vi "MH_T2HeaderInfo.vi"(8 "entrée d'erreur":errorcluster, 10 "CountRates":i32[](array[numeric]), 11 "InstrClass":refnum<class "MultiHarp150.lvclass"> caption="DNL_LabVIEW Object in") -> (0 "sortie d'erreur":errorcluster, 2 "HeaderTags":T1(array[cluster]))   [LabVIEW 2019, in "MultiHarp150.lvclass"]
uses:
  MultiHarp150.lvclass
  MultiHarp150.lvclass/MultiHarp150.ctl
panel:
  in  "BaseTagArray":T1(array[cluster])=[{"TagIdent"="File_GUID", "TagIndex"=-1, "TagType"=1073872895, "TagValue"=40, "TagAuxData"="{197B8EE0-02FE-45EA-A6B5-3F8BBDE2D882}\u0000\u0000"}, {"TagIdent"="File_AssuredContent", "TagIndex"=-1, "TagType"=1073872895, "TagValue"=32, "TagAuxData"="MultiHarp: HWSETG SWSETG\u0000\u0000\u0000\u0000\u0000\u0000\u0000\u0000"}, {"TagIdent"="CreatorSW_ContentVersion", "TagIndex"=-1, "TagType"=1073872895, "TagValue"=8, "TagAuxData"="1.0\u0000\u0000\u0000\u0000\u0000"}, {"TagIdent"="CreatorSW_Name", "TagIndex"=-1, "TagType"=1073872895, "TagValue"=16, "TagAuxData"="MultiHarp AcqUI\u0000"}, {"TagIdent"="CreatorSW_Version", "TagIndex"=-1, "TagType"=1073872895, "TagValue"=8, "TagAuxData"="3.0.0.0\u0000"}, {"TagIdent"="File_CreatingTime", "TagIndex"=-1, "TagType"=553648136, "TagValue"=4676398420989345414, "TagAuxData"=""}, {"TagIdent"="File_Comment", "TagIndex"=-1, "TagType"=1073872895, "TagValue"=8, "TagAuxData"="T2 Mode\u0000"}, {"TagIdent"="Measurement_Mode", "TagIndex"=-1, "TagType"=268435464, "TagValue"=2, "TagAuxData"=""}, {"TagIdent"="Measurement_SubMode", "TagIndex"=-1, "TagType"=268435464, "TagValue"=0, "TagAuxData"=""}, {"TagIdent"="TTResult_StopReason", "TagIndex"=-1, "TagType"=268435464, "TagValue"=0, "TagAuxData"=""}, {"TagIdent"="Fast_Load_End", "TagIndex"=-1, "TagType"=-65528, "TagValue"=0, "TagAuxData"=""}, {"TagIdent"="TTResultFormat_TTTRRecType", "TagIndex"=-1, "TagType"=268435464, "TagValue"=66055, "TagAuxData"=""}, {"TagIdent"="TTResultFormat_BitsPerRecord", "TagIndex"=-1, "TagType"=268435464, "TagValue"=32, "TagAuxData"=""}, {"TagIdent"="MeasDesc_BinningFactor", "TagIndex"=-1, "TagType"=268435464, "TagValue"=32, "TagAuxData"=""}, {"TagIdent"="MeasDesc_Offset", "TagIndex"=-1, "TagType"=268435464, "TagValue"=0, "TagAuxData"=""}, {"TagIdent"="MeasDesc_AcquisitionTime", "TagIndex"=-1, "TagType"=268435464, "TagValue"=900000, "TagAuxData"=""}, {"TagIdent"="MeasDesc_StopAt", "TagIndex"=-1, "TagType"=268435464, "TagValue"=4294967295, "TagAuxData"=""}, {"TagIdent"="MeasDesc_StopOnOvfl", "TagIndex"=-1, "TagType"=8, "TagValue"=0, "TagAuxData"=""}, {"TagIdent"="MeasDesc_Restart", "TagIndex"=-1, "TagType"=8, "TagValue"=0, "TagAuxData"=""}, {"TagIdent"="CurSWSetting_DispLog", "TagIndex"=-1, "TagType"=8, "TagValue"=-1, "TagAuxData"=""}, {"TagIdent"="CurSWSetting_DispAxisTimeFrom", "TagIndex"=-1, "TagType"=268435464, "TagValue"=1, "TagAuxData"=""}, {"TagIdent"="CurSWSetting_DispAxisTimeTo", "TagIndex"=-1, "TagType"=268435464, "TagValue"=120, "TagAuxData"=""}, {"TagIdent"="CurSWSetting_DispAxisCountFrom", "TagIndex"=-1, "TagType"=268435464, "TagValue"=1, "TagAuxData"=""}, {"TagIdent"="CurSWSetting_DispAxisCountTo", "TagIndex"=-1, "TagType"=268435464, "TagValue"=10000, "TagAuxData"=""}, {"TagIdent"="CurSWSetting_DispCurves", "TagIndex"=-1, "TagType"=268435464, "TagValue"=16, "TagAuxData"=""}, {"TagIdent"="CurSWSetting_DispCurve_MapTo", "TagIndex"=0, "TagType"=268435464, "TagValue"=0, "TagAuxData"=""}, {"TagIdent"="CurSWSetting_DispCurve_Show", "TagIndex"=0, "TagType"=8, "TagValue"=-1, "TagAuxData"=""}, {"TagIdent"="CurSWSetting_DispCurve_MapTo", "TagIndex"=1, "TagType"=268435464, "TagValue"=1, "TagAuxData"=""}, {"TagIdent"="CurSWSetting_DispCurve_Show", "TagIndex"=1, "TagType"=8, "TagValue"=-1, "TagAuxData"=""}, {"TagIdent"="CurSWSetting_DispCurve_MapTo", "TagIndex"=2, "TagType"=268435464, "TagValue"=2, "TagAuxData"=""}, {"TagIdent"="CurSWSetting_DispCurve_Show", "TagIndex"=2, "TagType"=8, "TagValue"=-1, "TagAuxData"=""}, {"TagIdent"="CurSWSetting_DispCurve_MapTo", "TagIndex"=3, "TagType"=268435464, "TagValue"=3, "TagAuxData"=""}, {"TagIdent"="CurSWSetting_DispCurve_Show", "TagIndex"=3, "TagType"=8, "TagValue"=-1, "TagAuxData"=""}, {"TagIdent"="CurSWSetting_DispCurve_MapTo", "TagIndex"=4, "TagType"=268435464, "TagValue"=4, "TagAuxData"=""}, {"TagIdent"="CurSWSetting_DispCurve_Show", "TagIndex"=4, "TagType"=8, "TagValue"=-1, "TagAuxData"=""}, {"TagIdent"="CurSWSetting_DispCurve_MapTo", "TagIndex"=5, "TagType"=268435464, "TagValue"=5, "TagAuxData"=""}, {"TagIdent"="CurSWSetting_DispCurve_Show", "TagIndex"=5, "TagType"=8, "TagValue"=-1, "TagAuxData"=""}, {"TagIdent"="CurSWSetting_DispCurve_MapTo", "TagIndex"=6, "TagType"=268435464, "TagValue"=6, "TagAuxData"=""}, {"TagIdent"="CurSWSetting_DispCurve_Show", "TagIndex"=6, "TagType"=8, "TagValue"=-1, "TagAuxData"=""}, {"TagIdent"="CurSWSetting_DispCurve_MapTo", "TagIndex"=7, "TagType"=268435464, "TagValue"=7, "TagAuxData"=""}, {"TagIdent"="CurSWSetting_DispCurve_Show", "TagIndex"=7, "TagType"=8, "TagValue"=-1, "TagAuxData"=""}, {"TagIdent"="CurSWSetting_DispCurve_MapTo", "TagIndex"=8, "TagType"=268435464, "TagValue"=8, "TagAuxData"=""}, {"TagIdent"="CurSWSetting_DispCurve_Show", "TagIndex"=8, "TagType"=8, "TagValue"=-1, "TagAuxData"=""}, {"TagIdent"="CurSWSetting_DispCurve_MapTo", "TagIndex"=9, "TagType"=268435464, "TagValue"=9, "TagAuxData"=""}, {"TagIdent"="CurSWSetting_DispCurve_Show", "TagIndex"=9, "TagType"=8, "TagValue"=-1, "TagAuxData"=""}, {"TagIdent"="CurSWSetting_DispCurve_MapTo", "TagIndex"=10, "TagType"=268435464, "TagValue"=10, "TagAuxData"=""}, {"TagIdent"="CurSWSetting_DispCurve_Show", "TagIndex"=10, "TagType"=8, "TagValue"=-1, "TagAuxData"=""}, {"TagIdent"="CurSWSetting_DispCurve_MapTo", "TagIndex"=11, "TagType"=268435464, "TagValue"=11, "TagAuxData"=""}, {"TagIdent"="CurSWSetting_DispCurve_Show", "TagIndex"=11, "TagType"=8, "TagValue"=-1, "TagAuxData"=""}, {"TagIdent"="CurSWSetting_DispCurve_MapTo", "TagIndex"=12, "TagType"=268435464, "TagValue"=12, "TagAuxData"=""}, {"TagIdent"="CurSWSetting_DispCurve_Show", "TagIndex"=12, "TagType"=8, "TagValue"=-1, "TagAuxData"=""}, {"TagIdent"="CurSWSetting_DispCurve_MapTo", "TagIndex"=13, "TagType"=268435464, "TagValue"=13, "TagAuxData"=""}, {"TagIdent"="CurSWSetting_DispCurve_Show", "TagIndex"=13, "TagType"=8, "TagValue"=-1, "TagAuxData"=""}, {"TagIdent"="CurSWSetting_DispCurve_MapTo", "TagIndex"=14, "TagType"=268435464, "TagValue"=14, "TagAuxData"=""}, {"TagIdent"="CurSWSetting_DispCurve_Show", "TagIndex"=14, "TagType"=8, "TagValue"=-1, "TagAuxData"=""}, {"TagIdent"="CurSWSetting_DispCurve_MapTo", "TagIndex"=15, "TagType"=268435464, "TagValue"=15, "TagAuxData"=""}, {"TagIdent"="CurSWSetting_DispCurve_Show", "TagIndex"=15, "TagType"=8, "TagValue"=-1, "TagAuxData"=""}, {"TagIdent"="HW_Type", "TagIndex"=-1, "TagType"=1073872895, "TagValue"=24, "TagAuxData"="MultiHarp 150 4P\u0000\u0000\u0000\u0000\u0000\u0000\u0000\u0000"}, {"TagIdent"="HW_PartNo", "TagIndex"=-1, "TagType"=1073872895, "TagValue"=8, "TagAuxData"="930043\u0000\u0000"}, {"TagIdent"="HW_Version", "TagIndex"=-1, "TagType"=1073872895, "TagValue"=8, "TagAuxData"="1.0\u0000\u0000\u0000\u0000\u0000"}, {"TagIdent"="HW_SerialNo", "TagIndex"=-1, "TagType"=1073872895, "TagValue"=8, "TagAuxData"="1043897\u0000"}, {"TagIdent"="HW_Features", "TagIndex"=-1, "TagType"=285212680, "TagValue"=183, "TagAuxData"=""}, {"TagIdent"="HW_BaseResolution", "TagIndex"=-1, "TagType"=536870920, "TagValue"=4437731733528994965, "TagAuxData"=""}, {"TagIdent"="HW_InpChannels", "TagIndex"=-1, "TagType"=268435464, "TagValue"=4, "TagAuxData"=""}, {"TagIdent"="HW_ExternalRefClock", "TagIndex"=-1, "TagType"=8, "TagValue"=0, "TagAuxData"=""}, {"TagIdent"="HW_ExternalDevices", "TagIndex"=-1, "TagType"=268435464, "TagValue"=0, "TagAuxData"=""}, {"TagIdent"="HWTriggerOut_Period", "TagIndex"=-1, "TagType"=536870920, "TagValue"=4502148214488346441, "TagAuxData"=""}, {"TagIdent"="HWTriggerOut_On", "TagIndex"=-1, "TagType"=8, "TagValue"=0, "TagAuxData"=""}, {"TagIdent"="HW_InputHysteresis", "TagIndex"=-1, "TagType"=8, "TagValue"=0, "TagAuxData"=""}, {"TagIdent"="HWSync_Divider", "TagIndex"=-1, "TagType"=268435464, "TagValue"=1, "TagAuxData"=""}, {"TagIdent"="HWSync_TrgLevel", "TagIndex"=-1, "TagType"=268435464, "TagValue"=-10, "TagAuxData"=""}, {"TagIdent"="HWSync_TrgEdge", "TagIndex"=-1, "TagType"=268435464, "TagValue"=0, "TagAuxData"=""}, {"TagIdent"="HWSync_Offset", "TagIndex"=-1, "TagType"=268435464, "TagValue"=27000, "TagAuxData"=""}, {"TagIdent"="HWSync_TdCode", "TagIndex"=-1, "TagType"=268435464, "TagValue"=0, "TagAuxData"=""}, {"TagIdent"="HWInpChan_TrgLevel", "TagIndex"=0, "TagType"=268435464, "TagValue"=-150, "TagAuxData"=""}, {"TagIdent"="HWInpChan_TrgEdge", "TagIndex"=0, "TagType"=268435464, "TagValue"=0, "TagAuxData"=""}, {"TagIdent"="HWInpChan_Offset", "TagIndex"=0, "TagType"=268435464, "TagValue"=0, "TagAuxData"=""}, {"TagIdent"="HWInpChan_Enabled", "TagIndex"=0, "TagType"=8, "TagValue"=-1, "TagAuxData"=""}, {"TagIdent"="HWInpChan_TdCode", "TagIndex"=0, "TagType"=268435464, "TagValue"=0, "TagAuxData"=""}, {"TagIdent"="HWInpChan_TrgLevel", "TagIndex"=1, "TagType"=268435464, "TagValue"=-150, "TagAuxData"=""}, {"TagIdent"="HWInpChan_TrgEdge", "TagIndex"=1, "TagType"=268435464, "TagValue"=0, "TagAuxData"=""}, {"TagIdent"="HWInpChan_Offset", "TagIndex"=1, "TagType"=268435464, "TagValue"=0, "TagAuxData"=""}, {"TagIdent"="HWInpChan_Enabled", "TagIndex"=1, "TagType"=8, "TagValue"=-1, "TagAuxData"=""}, {"TagIdent"="HWInpChan_TdCode", "TagIndex"=1, "TagType"=268435464, "TagValue"=0, "TagAuxData"=""}, {"TagIdent"="HWInpChan_TrgLevel", "TagIndex"=2, "TagType"=268435464, "TagValue"=-50, "TagAuxData"=""}, {"TagIdent"="HWInpChan_TrgEdge", "TagIndex"=2, "TagType"=268435464, "TagValue"=0, "TagAuxData"=""}, {"TagIdent"="HWInpChan_Offset", "TagIndex"=2, "TagType"=268435464, "TagValue"=0, "TagAuxData"=""}, {"TagIdent"="HWInpChan_Enabled", "TagIndex"=2, "TagType"=8, "TagValue"=-1, "TagAuxData"=""}, {"TagIdent"="HWInpChan_TdCode", "TagIndex"=2, "TagType"=268435464, "TagValue"=0, "TagAuxData"=""}, {"TagIdent"="HWInpChan_TrgLevel", "TagIndex"=3, "TagType"=268435464, "TagValue"=-50, "TagAuxData"=""}, {"TagIdent"="HWInpChan_TrgEdge", "TagIndex"=3, "TagType"=268435464, "TagValue"=0, "TagAuxData"=""}, {"TagIdent"="HWInpChan_Offset", "TagIndex"=3, "TagType"=268435464, "TagValue"=0, "TagAuxData"=""}, {"TagIdent"="HWInpChan_Enabled", "TagIndex"=3, "TagType"=8, "TagValue"=-1, "TagAuxData"=""}, {"TagIdent"="HWInpChan_TdCode", "TagIndex"=3, "TagType"=268435464, "TagValue"=0, "TagAuxData"=""}, {"TagIdent"="MeasDesc_Resolution", "TagIndex"=-1, "TagType"=536870920, "TagValue"=4437731733528994965, "TagAuxData"=""}, {"TagIdent"="HW_Markers", "TagIndex"=-1, "TagType"=268435464, "TagValue"=4, "TagAuxData"=""}, {"TagIdent"="HWMarkers_RisingEdge", "TagIndex"=0, "TagType"=8, "TagValue"=0, "TagAuxData"=""}, {"TagIdent"="HWMarkers_RisingEdge", "TagIndex"=1, "TagType"=8, "TagValue"=0, "TagAuxData"=""}, {"TagIdent"="HWMarkers_RisingEdge", "TagIndex"=2, "TagType"=8, "TagValue"=0, "TagAuxData"=""}, {"TagIdent"="HWMarkers_RisingEdge", "TagIndex"=3, "TagType"=8, "TagValue"=0, "TagAuxData"=""}, {"TagIdent"="HWMarkers_Enabled", "TagIndex"=0, "TagType"=8, "TagValue"=-1, "TagAuxData"=""}, {"TagIdent"="HWMarkers_Enabled", "TagIndex"=1, "TagType"=8, "TagValue"=-1, "TagAuxData"=""}, {"TagIdent"="HWMarkers_Enabled", "TagIndex"=2, "TagType"=8, "TagValue"=-1, "TagAuxData"=""}, {"TagIdent"="HWMarkers_Enabled", "TagIndex"=3, "TagType"=8, "TagValue"=-1, "TagAuxData"=""}, {"TagIdent"="HWMarkers_HoldOff", "TagIndex"=-1, "TagType"=268435464, "TagValue"=0, "TagAuxData"=""}, {"TagIdent"="MeasDesc_GlobalResolution", "TagIndex"=-1, "TagType"=536870920, "TagValue"=4437731733528994965, "TagAuxData"=""}, {"TagIdent"="TTResult_SyncRate", "TagIndex"=-1, "TagType"=268435464, "TagValue"=0, "TagAuxData"=""}, {"TagIdent"="TTResult_InputRate", "TagIndex"=0, "TagType"=268435464, "TagValue"=9126, "TagAuxData"=""}, {"TagIdent"="TTResult_InputRate", "TagIndex"=1, "TagType"=268435464, "TagValue"=8247, "TagAuxData"=""}, {"TagIdent"="TTResult_InputRate", "TagIndex"=2, "TagType"=268435464, "TagValue"=0, "TagAuxData"=""}, {"TagIdent"="TTResult_InputRate", "TagIndex"=3, "TagType"=268435464, "TagValue"=0, "TagAuxData"=""}, {"TagIdent"="TTResult_StopAfter", "TagIndex"=-1, "TagType"=268435464, "TagValue"=900000, "TagAuxData"=""}, {"TagIdent"="TTResult_NumberOfRecords", "TagIndex"=-1, "TagType"=268435464, "TagValue"=10000, "TagAuxData"=""}, {"TagIdent"="TTResult_MDescWarningFlags", "TagIndex"=-1, "TagType"=285212680, "TagValue"=0, "TagAuxData"=""}, {"TagIdent"="Header_End", "TagIndex"=-1, "TagType"=-65528, "TagValue"=0, "TagAuxData"=""}] {"TagType" format="%x"}
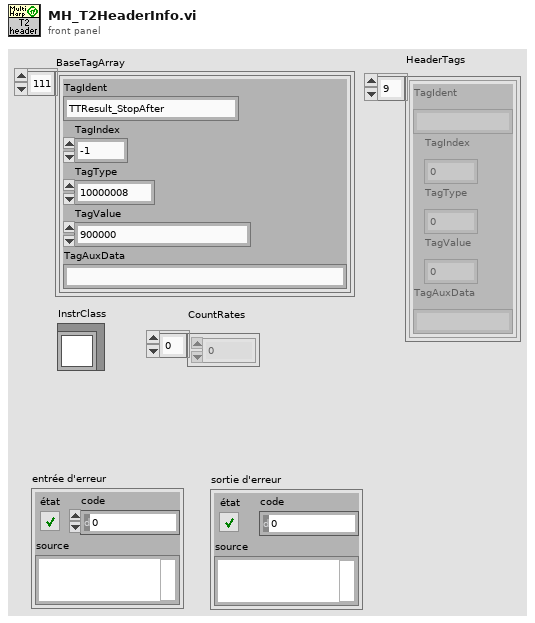
[diagram p1: front panel]
types:
  T1 = cluster{"TagIdent":string, "TagIndex":i32, "TagType":i32, "TagValue":i64, "TagAuxData":string}[]
  T2 = cluster{"TagIdent":string, "TagIndex":i32, "TagType":i32, "TagValue":i64, "TagAuxData":string}
  T3 = enum16{"5", "10", "20", "40", "80", "160", "320", "640", "1280", "2560", "5120", "10240", "20480", "40960", "81920", "163840", "327680", "655360", "1310720", "2621440", "5242880", "10485760", "20971520", "41943040"}
  T4 = typedef "MH_InputChannel_LS.ctl" = cluster{"Name":string, "Enable":bool, "Edge":i32, "Level":i32, "Offset":i32, "UseDeadTime":bool, "DeadTime":i32}
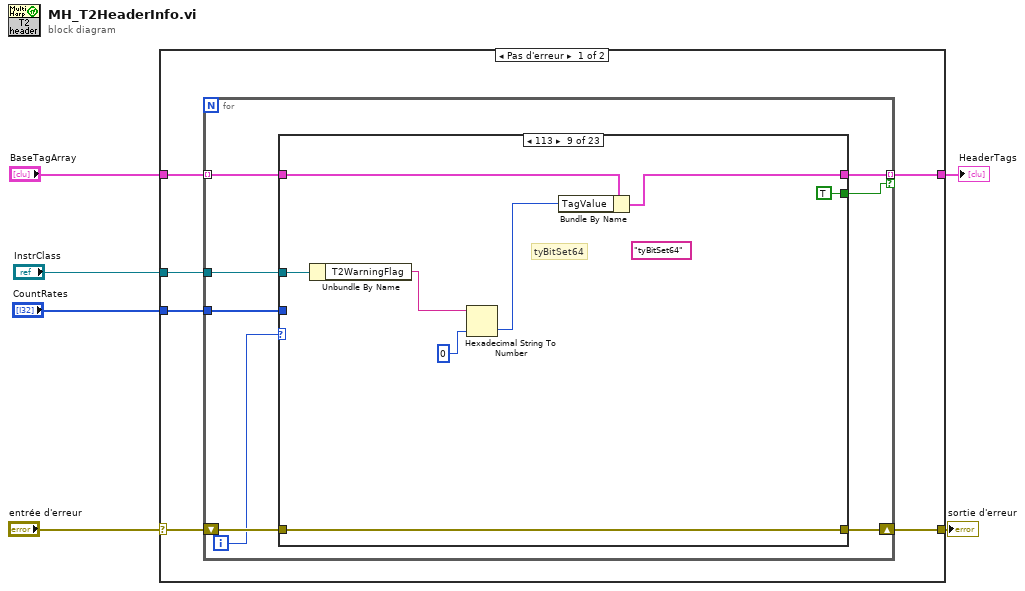
[diagram p0: block diagram]
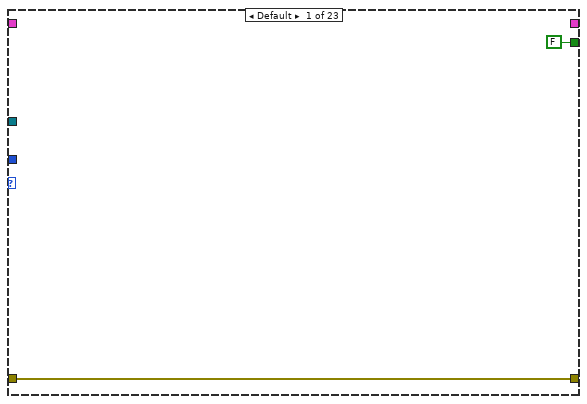
[diagram p2: hidden frame]
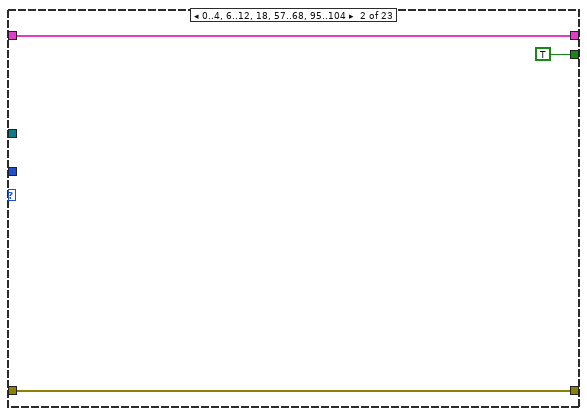
[diagram p3: hidden frame]
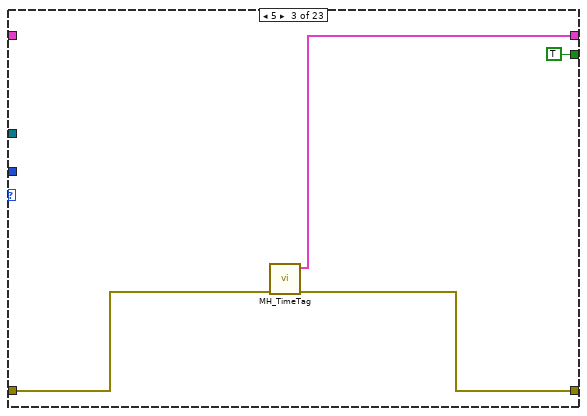
[diagram p4: hidden frame]
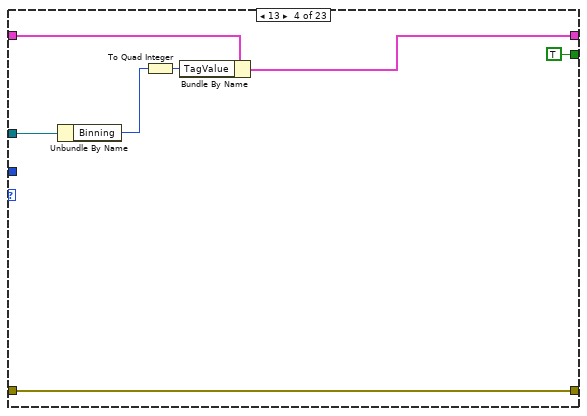
[diagram p5: hidden frame]
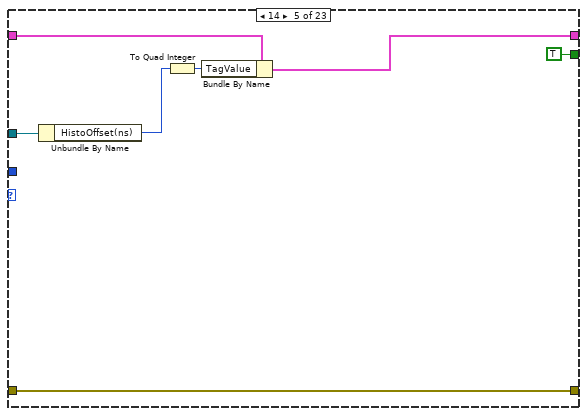
[diagram p6: hidden frame]
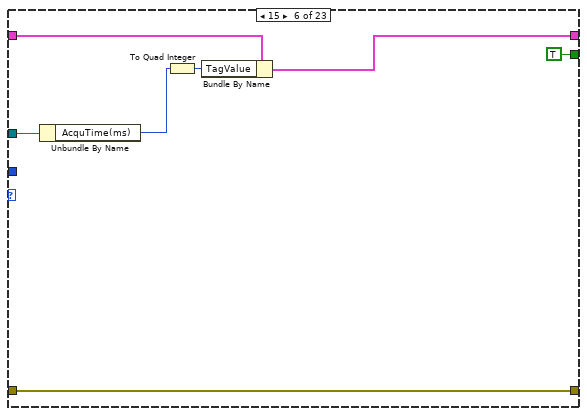
[diagram p7: hidden frame]
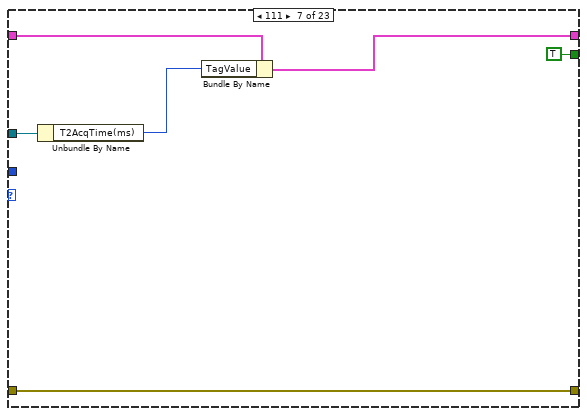
[diagram p8: hidden frame]
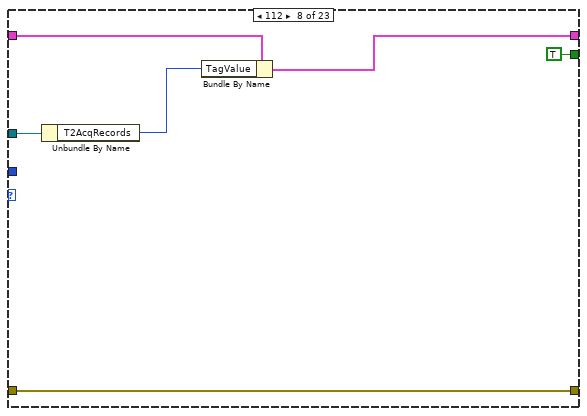
[diagram p9: hidden frame]
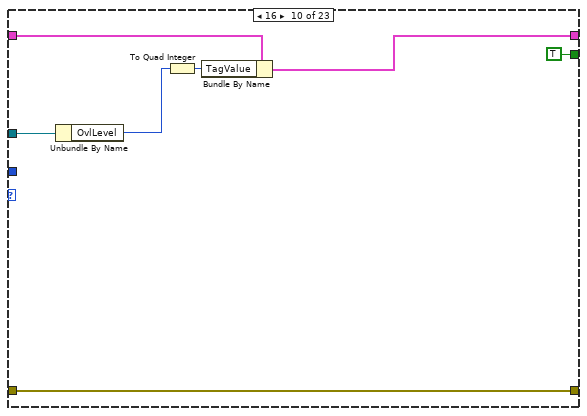
[diagram p10: hidden frame]
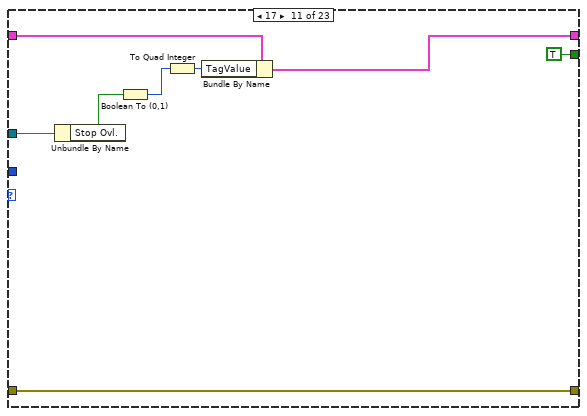
[diagram p11: hidden frame]
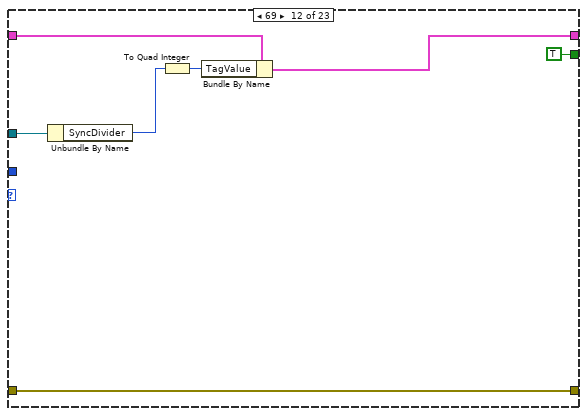
[diagram p12: hidden frame]
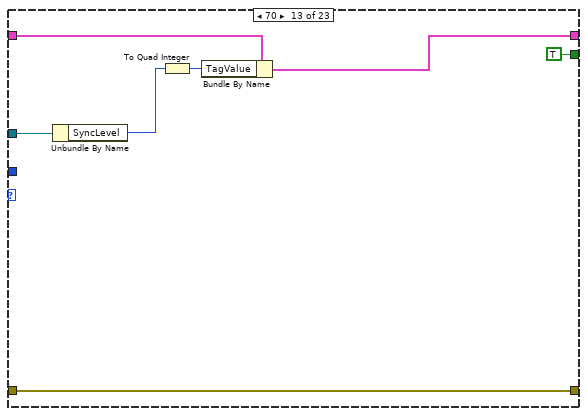
[diagram p13: hidden frame]
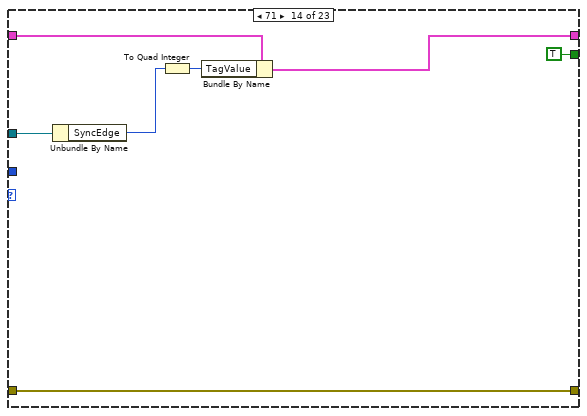
[diagram p14: hidden frame]
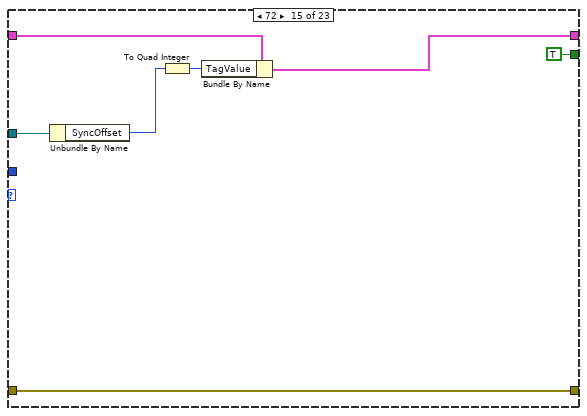
[diagram p15: hidden frame]
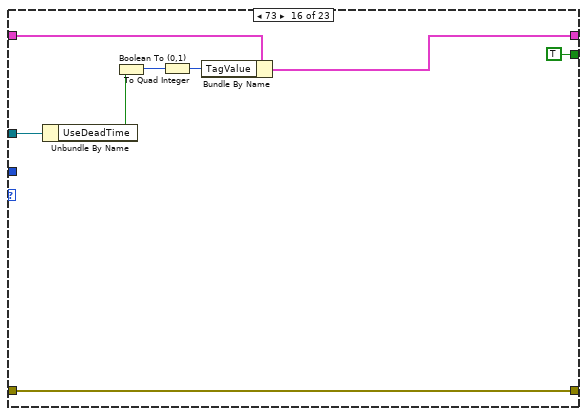
[diagram p16: hidden frame]
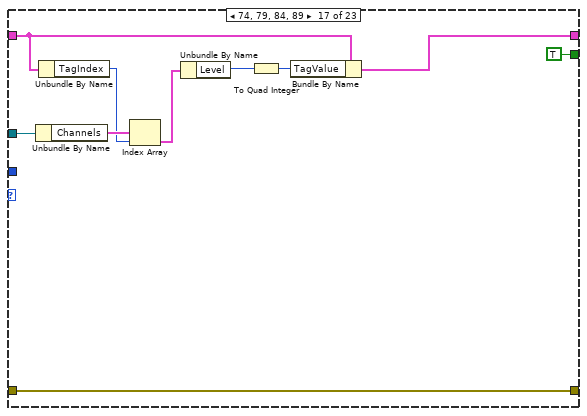
[diagram p17: hidden frame]
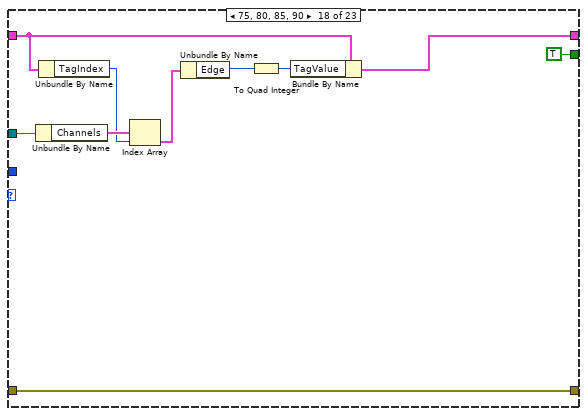
[diagram p18: hidden frame]
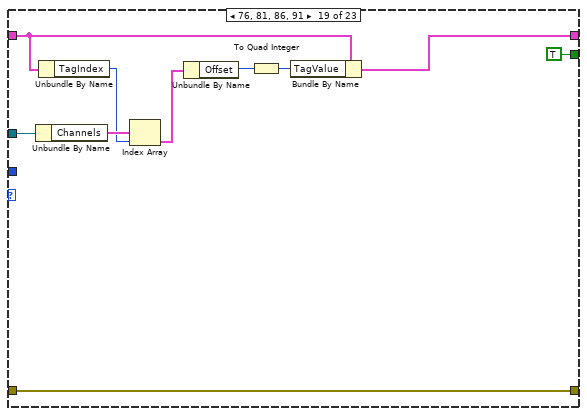
[diagram p19: hidden frame]
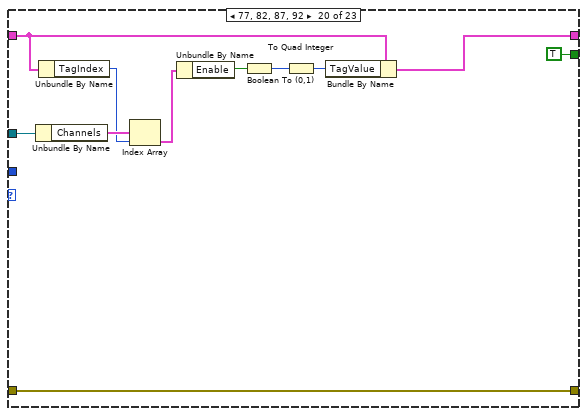
[diagram p20: hidden frame]
diagram:
  n1 = case shown="Pas d'erreur" "entrée d'erreur" {
    selector: "entrée d'erreur" -> [w11 w198]
    tunnel: [w12 w198] -> w6
    tunnel: "BaseTagArray" -> [w10 _]
    tunnel: "InstrClass" -> [w9 _]
    tunnel: [w8 _] -> w2
    tunnel: "CountRates" -> [w7 _]
    frame No Error {
      n2 = for {
        shift-right: [w20] -> w12
        shift-left: w11 -> [w19]
        tunnel: w10 -> [w14] mode=indexing
        tunnel: [w17] -> w8 mode=indexing if=w15
        tunnel: w9 -> [w16]
        tunnel: w7 -> [w13]
        i -> [w18]
        n3 = case shown="113" w18 {
          selector: w18 -> [_ _ _ _ _ _ _ _ _ _ _ _ _ _ _ _ _ _ _ _ _ _ w190]
          tunnel: [w22 w24 w29 w31 w38 w46 w53 w59 w67 w72 w81 w88 w95 w102 w109 w117 w128 w138 w148 w159 w170 w185 w196] -> w20
          tunnel: w19 -> [w22 w24 w28 w31 w38 w46 w53 w59 w67 w72 w81 w88 w95 w102 w109 w117 w128 w138 w148 w159 w170 w185 w196]
          tunnel: w14 -> [_ w25 _ w35 w42 w49 w55 w61 w69 w76 w84 w91 w98 w105 w112 w120 w123 w133 w143 w154 w165 w183 w194]
          tunnel: [_ w25 w27 w33 w40 w48 w54 w60 w68 w74 w83 w90 w97 w104 w111 w119 w130 w140 w150 w161 w172 w186 w197] -> w17
          tunnel: w16 -> [_ _ _ w36 w43 w50 w56 w62 w70 w77 w85 w92 w99 w106 w113 w121 w131 w141 w151 w162 w173 w187 _]
          tunnel: [FALSE TRUE TRUE TRUE TRUE TRUE TRUE TRUE TRUE TRUE TRUE TRUE TRUE TRUE TRUE TRUE TRUE TRUE TRUE TRUE TRUE TRUE TRUE] -> w15
          tunnel: w13 -> [_ _ _ _ _ _ _ _ _ _ _ _ _ _ _ _ _ _ _ _ _ _ w193]
          frame Default {
          }
          frame 0..4, 6..12, 18, 57..68, 95..104 {
          }
          frame 5 {
            n4 = call <userlib>:"MH_TimeTag.vi"("entrée d'erreur"=w28) -> ("sortie d'erreur"=w29:errorcluster, "TimeTag"=w27:T2)  [unwired: 8 in, 1 out]
          }
          frame 13 {
            n5 = Unbundle By Name(w36) -> ("Binning"=w34:T3)
            n6 = To Quad Integer(1:w34) -> (0:w32:i64)
            n7 = Bundle By Name(cluster=w35, "TagValue"=w32) -> (w33:T2)
          }
          frame 14 {
            n8 = Unbundle By Name(w43) -> ("HistoOffset(ns)"=w41:i32)
            n9 = To Quad Integer(1:w41) -> (0:w39:i64)
            n10 = Bundle By Name(cluster=w42, "TagValue"=w39) -> (w40:T2)
          }
          frame 15 {
            n11 = Unbundle By Name(w50) -> ("AcquTime(ms)"=w44:i32)
            n12 = To Quad Integer(1:w44) -> (0:w47:i64)
            n13 = Bundle By Name(cluster=w49, "TagValue"=w47) -> (w48:T2)
          }
          frame 111 {
            n14 = Unbundle By Name(w56) -> ("T2AcqTime(ms)"=w51:i64)
            n15 = Bundle By Name(cluster=w55, "TagValue"=w51) -> (w54:T2)
          }
          frame 112 {
            n16 = Unbundle By Name(w62) -> ("T2AcqRecords"=w57:i64)
            n17 = Bundle By Name(cluster=w61, "TagValue"=w57) -> (w60:T2)
          }
          frame 113 {
            (unwired) "tyBitSet64" ("string")
            # "tyBitSet64"
            n18 = Unbundle By Name(w70) -> ("T2WarningFlag"=w63:string)
            n19 = Hexadecimal String To Number(string=w63, default (0uL)=i64 0 ("TagValue")) -> (number=w64:i64)  [unwired: 1 in, 1 out]
            n20 = Bundle By Name(cluster=w69, "TagValue"=w64) -> (w68:T2)
          }
          frame 16 {
            n21 = Unbundle By Name(w77) -> ("OvlLevel"=w75:u32)
            n22 = To Quad Integer(1:w75) -> (0:w73:i64)
            n23 = Bundle By Name(cluster=w76, "TagValue"=w73) -> (w74:T2)
          }
          frame 17 {
            n24 = Unbundle By Name(w85) -> ("Stop Ovl."=w80:bool)
            n25 = Boolean To (0,1)(Boolean=w80) -> (0, 1=w79:i16)
            n26 = To Quad Integer(1:w79) -> (0:w82:i64)
            n27 = Bundle By Name(cluster=w84, "TagValue"=w82) -> (w83:T2)
          }
          frame 69 {
            n28 = Unbundle By Name(w92) -> ("SyncDivider"=w86:i32)
            n29 = To Quad Integer(1:w86) -> (0:w89:i64)
            n30 = Bundle By Name(cluster=w91, "TagValue"=w89) -> (w90:T2)
          }
          frame 70 {
            n31 = Unbundle By Name(w99) -> ("SyncLevel"=w93:i32)
            n32 = To Quad Integer(1:w93) -> (0:w96:i64)
            n33 = Bundle By Name(cluster=w98, "TagValue"=w96) -> (w97:T2)
          }
          frame 71 {
            n34 = Unbundle By Name(w106) -> ("SyncEdge"=w100:i32)
            n35 = To Quad Integer(1:w100) -> (0:w103:i64)
            n36 = Bundle By Name(cluster=w105, "TagValue"=w103) -> (w104:T2)
          }
          frame 72 {
            n37 = Unbundle By Name(w113) -> ("SyncOffset"=w107:i32)
            n38 = To Quad Integer(1:w107) -> (0:w110:i64)
            n39 = Bundle By Name(cluster=w112, "TagValue"=w110) -> (w111:T2)
          }
          frame 73 {
            n40 = Unbundle By Name(w121) -> ("UseDeadTime"=w115:bool)
            n41 = Boolean To (0,1)(Boolean=w115) -> (0, 1=w114:i16)
            n42 = To Quad Integer(1:w114) -> (0:w118:i64)
            n43 = Bundle By Name(cluster=w120, "TagValue"=w118) -> (w119:T2)
          }
          frame 74, 79, 84, 89 {
            n44 = Unbundle By Name(w131) -> ("Channels"=w126:T4[])
            n45 = Unbundle By Name(w123) -> ("TagIndex"=w122:i32)
            n46 = Index Array(array=w126, index=w122) -> (element=w124:T4)
            n47 = Unbundle By Name(w124) -> ("Level"=w125:i32)
            n48 = To Quad Integer(1:w125) -> (0:w129:i64)
            n49 = Bundle By Name(cluster=w123, "TagValue"=w129) -> (w130:T2)
          }
          frame 75, 80, 85, 90 {
            n50 = Unbundle By Name(w141) -> ("Channels"=w136:T4[])
            n51 = Unbundle By Name(w133) -> ("TagIndex"=w132:i32)
            n52 = Index Array(array=w136, index=w132) -> (element=w134:T4)
            n53 = Unbundle By Name(w134) -> ("Edge"=w135:i32)
            n54 = To Quad Integer(1:w135) -> (0:w139:i64)
            n55 = Bundle By Name(cluster=w133, "TagValue"=w139) -> (w140:T2)
          }
          frame 76, 81, 86, 91 {
            n56 = Unbundle By Name(w151) -> ("Channels"=w146:T4[])
            n57 = Unbundle By Name(w143) -> ("TagIndex"=w142:i32)
            n58 = Index Array(array=w146, index=w142) -> (element=w144:T4)
            n59 = Unbundle By Name(w144) -> ("Offset"=w145:i32)
            n60 = To Quad Integer(1:w145) -> (0:w149:i64)
            n61 = Bundle By Name(cluster=w143, "TagValue"=w149) -> (w150:T2)
          }
          frame 77, 82, 87, 92 {
            n62 = Unbundle By Name(w162) -> ("Channels"=w157:T4[])
            n63 = Unbundle By Name(w154) -> ("TagIndex"=w153:i32)
            n64 = Index Array(array=w157, index=w153) -> (element=w155:T4)
            n65 = Unbundle By Name(w155) -> ("Enable"=w156:bool)
            n66 = Boolean To (0,1)(Boolean=w156) -> (0, 1=w152:i16)
            n67 = To Quad Integer(1:w152) -> (0:w160:i64)
            n68 = Bundle By Name(cluster=w154, "TagValue"=w160) -> (w161:T2)
          }
          frame 78, 83, 88, 93 {
            n69 = Unbundle By Name(w173) -> ("Channels"=w168:T4[])
            n70 = Unbundle By Name(w165) -> ("TagIndex"=w164:i32)
            n71 = Index Array(array=w168, index=w164) -> (element=w166:T4)
            n72 = Unbundle By Name(w166) -> ("UseDeadTime"=w167:bool)
            n73 = Boolean To (0,1)(Boolean=w167) -> (0, 1=w163:i16)
            n74 = To Quad Integer(1:w163) -> (0:w171:i64)
            n75 = Bundle By Name(cluster=w165, "TagValue"=w171) -> (w172:T2)
          }
          frame 94, 105 {
            n76 = Unbundle By Name(w187) -> ("Binning"=w182:T3, "Resolution (ns)"=w181:dbl)
            n77 = Increment(x=w182) -> (x+1=w176:T3)
            n78 = To Double Precision Float(number=w176) -> (double precision float=w180:dbl)
            n79 = Multiply(x=w180, y=w181) -> (x*y=w179:dbl)
            n80 = Divide(x=w179, y=1000000000.0) -> (x/y=w175:dbl)
            n81 = Type Cast(type=i64 0, x=w175) -> (*(type *) &x=w178:i64)
            n82 = Bundle By Name(cluster=w183, "TagValue"=w178) -> (w186:T2)
          }
          frame 106..110 {
            n83 = Subtract(x=w190, y=106) -> (x-y=w188:i32)
            n84 = Index Array(array=w193, index=w188) -> (element=w192:i32)
            n85 = To Quad Integer(1:w192) -> (0:w191:i64)
            n86 = Bundle By Name(cluster=w194, "TagValue"=w191) -> (w197:T2)
          }
        }
      }
    }
    frame Error {
    }
  }
  "sortie d'erreur" <- w6
  "HeaderTags" <- w2
